vi "TransformColor.vi"(11 "Current Robot Sensor Color":T1) -> (3 "Next Field Sensor Color":T1)   [LabVIEW 2019]
uses:
  Controls/Colors.ctl
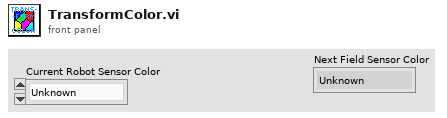
[diagram p1: front panel]
types:
  T1 = typedef "Colors.ctl" = enum16{"Unknown", "Yellow", "Red", "Green", "Blue"}
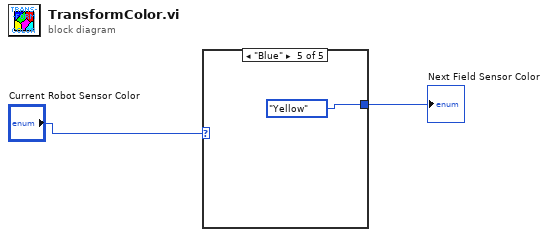
[diagram p0: block diagram]
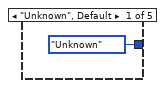
[diagram p2: hidden frame]
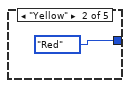
[diagram p3: hidden frame]
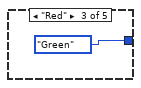
[diagram p4: hidden frame]
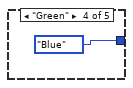
[diagram p5: hidden frame]
diagram:
  n1 = case shown="\"Blue\"" "Current Robot Sensor Color" {
    tunnel: [Colors."Unknown" ("Stop On Robot Sensor Color") Colors."Red" ("Stop On Robot Sensor Color") Colors."Green" ("Stop On Robot Sensor Color") Colors."Blue" ("Stop On Robot Sensor Color") Colors."Yellow" ("Stop On Robot Sensor Color")] -> w1
    frame "Unknown", Default {
    }
    frame "Yellow" {
    }
    frame "Red" {
    }
    frame "Green" {
    }
    frame "Blue" {
    }
  }
  "Next Field Sensor Color" <- w1
